vi "Boolean Update - Colors.vi"(6 "control-level":string, 10 "Bool Refnum":refnum<vi>, 11 "Material-Scheme in":refnum<class "Material-Scheme.lvclass">) -> (0 "error out":errorcluster, 1 "Array":cluster{"bg":u32, "fg":u32}[](array[cluster]), 2 "font color":u32(colorbox), 3 "Material-Scheme":refnum<class "Material-Scheme.lvclass">)   [LabVIEW 2021, in "TSC Material Theme.lvlib" / "Material-Scheme.lvclass"]
doc: "update boolean control colors\n\n<b>Code Developed By:</b>\nTechnology Service Corporation\nwww.tsc.com/atcs\n\nDeveloper:\nDaniel Coons"
uses:
  Material-Scheme.lvclass
  Material-Scheme.lvclass/Material-Scheme.ctl
panel:
  in  "error in":errorcluster
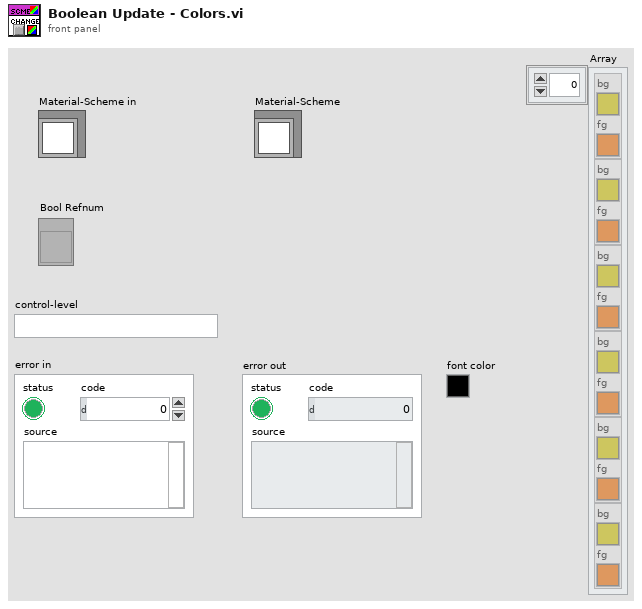
[diagram p1: front panel]
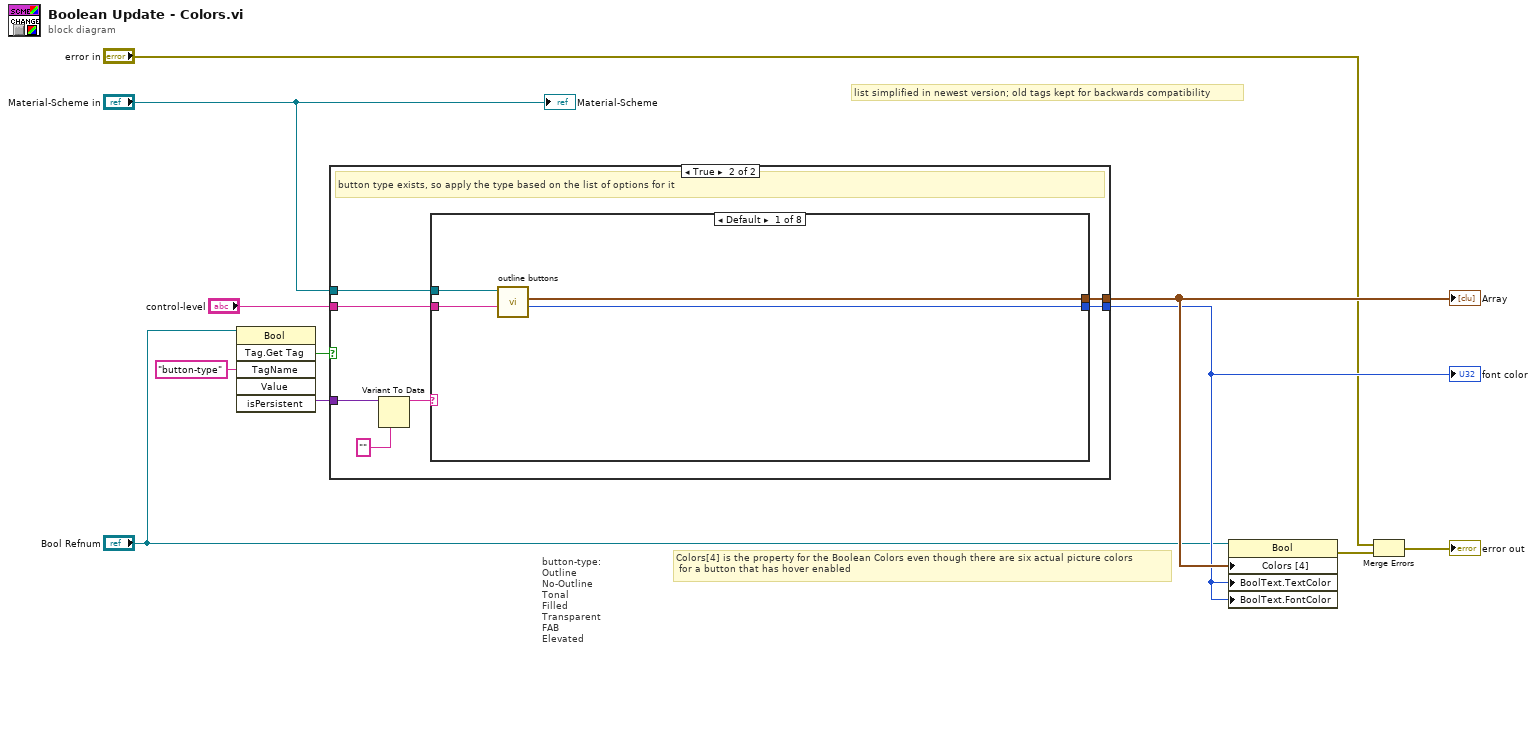
[diagram p0: block diagram]
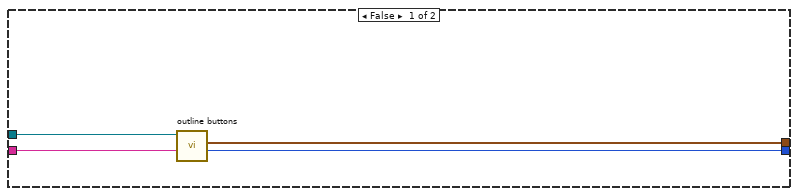
[diagram p2: hidden frame]
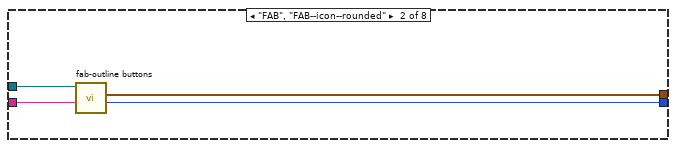
[diagram p3: hidden frame]
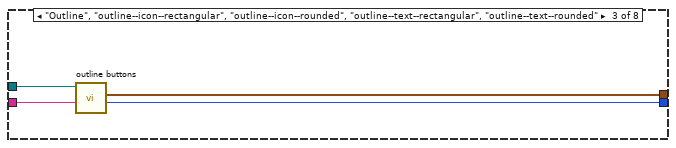
[diagram p4: hidden frame]
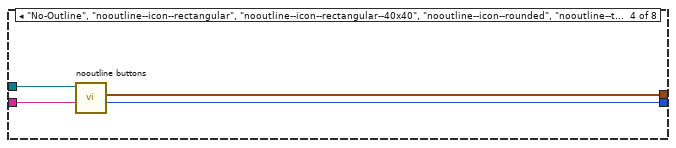
[diagram p5: hidden frame]
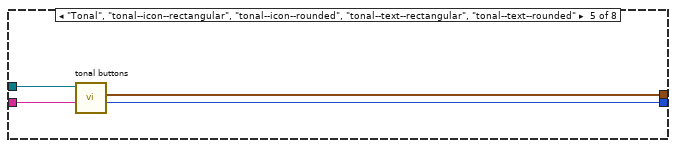
[diagram p6: hidden frame]
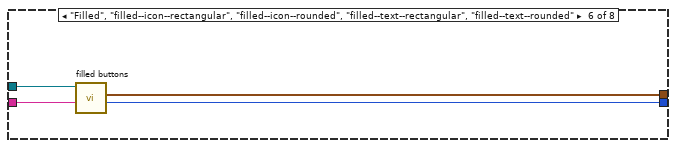
[diagram p7: hidden frame]
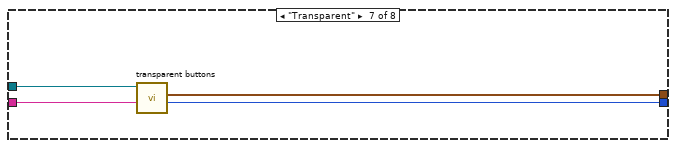
[diagram p8: hidden frame]
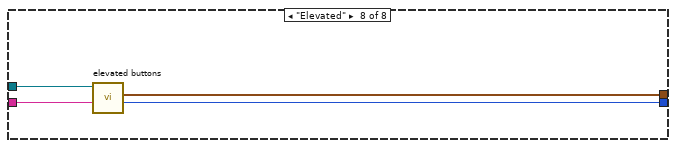
[diagram p9: hidden frame]
diagram:
  # "list simplified in newest version; old tags kept for backwards compatibility"
  # "button-type:\nOutline\nNo-Outline\nTonal\nFilled\nTransparent\nFAB\nElevated"
  # "Colors[4] is the property for the Boolean Colors even though there are six actual picture colors\n for a button that has hover enabled"
  n1 = invoke class="Bool" method="Tag.Get Tag"(reference="Bool Refnum", "TagName"="button-type" ("Tag Name")) -> ("GetTag"=w10:bool, "isPersistent"=w9:variant)  [unwired: 4 in, 4 out]
  n2 = case shown="True" w10 {
    tunnel: w9 -> [_ w22]
    tunnel: [w14 w19] -> w8
    tunnel: [w13 w18] -> w7
    tunnel: "Material-Scheme in" -> [w15 w17]
    tunnel: "control-level" -> [w12 w16]
    frame False {
      n3 = call "outline buttons.vi"("control-level"=w12, "Material-Scheme in"=w15) -> ("font color"=w13:u32, "colors array"=w14:cluster{"bg":u32, "fg":u32}[])  [unwired: 8 in]
    }
    frame True {
      # "button type exists, so apply the type based on the list of options for it"
      n4 = Variant To Data(type="", Variant=w22) -> (data=w20:string)  [unwired: 1 in, 1 out]
      n5 = case shown="Default" w20 {
        tunnel: [w26 w30 w34 w38 w42 w46 w48 w52] -> w19
        tunnel: [w25 w29 w33 w37 w41 w45 w47 w51] -> w18
        tunnel: w17 -> [w24 w28 w32 w36 w40 w44 w50 w54]
        tunnel: w16 -> [w23 w27 w31 w35 w39 w43 w49 w53]
        frame Default {
          n6 = call "outline buttons.vi"("control-level"=w23, "Material-Scheme in"=w24) -> ("font color"=w25:u32, "colors array"=w26:cluster{"bg":u32, "fg":u32}[])  [unwired: 8 in]
        }
        frame "FAB", "FAB--icon--rounded" {
          n7 = call "fab-outline buttons.vi"("control-level"=w27, "Material-Scheme in"=w28) -> ("font color"=w29:u32, "colors array"=w30:cluster{"bg":u32, "fg":u32}[])  [unwired: 8 in]
        }
        frame "Outline", "outline--icon--rectangular", "outline--icon--rounded", "outline--text--rectangular", "outline--text--rounded" {
          n8 = call "outline buttons.vi"("control-level"=w31, "Material-Scheme in"=w32) -> ("font color"=w33:u32, "colors array"=w34:cluster{"bg":u32, "fg":u32}[])  [unwired: 8 in]
        }
        frame "No-Outline", "nooutline--icon--rectangular", "nooutline--icon--rectangular--40x40", "nooutline--icon--rounded", "nooutline--text--rectangular", "nooutline--text--rounded" {
          n9 = call "nooutline buttons.vi"("control-level"=w35, "Material-Scheme in"=w36) -> ("font color"=w37:u32, "colors array"=w38:cluster{"bg":u32, "fg":u32}[])  [unwired: 8 in]
        }
        frame "Tonal", "tonal--icon--rectangular", "tonal--icon--rounded", "tonal--text--rectangular", "tonal--text--rounded" {
          n10 = call "tonal buttons.vi"("control-level"=w39, "Material-Scheme in"=w40) -> ("font color"=w41:u32, "colors array"=w42:cluster{"bg":u32, "fg":u32}[])  [unwired: 8 in]
        }
        frame "Filled", "filled--icon--rectangular", "filled--icon--rounded", "filled--text--rectangular", "filled--text--rounded" {
          n11 = call "filled buttons.vi"("control-level"=w43, "Material-Scheme in"=w44) -> ("font color"=w45:u32, "colors array"=w46:cluster{"bg":u32, "fg":u32}[])  [unwired: 8 in]
        }
        frame "Transparent" {
          n12 = call "transparent buttons.vi"("control-level"=w49, "Material-Scheme in"=w50) -> ("font color"=w47:u32, "colors array"=w48:cluster{"bg":u32, "fg":u32}[])  [unwired: 8 in]
        }
        frame "Elevated" {
          n13 = call "elevated buttons.vi"("control-level"=w53, "Material-Scheme in"=w54) -> ("font color"=w51:u32, "colors array"=w52:cluster{"bg":u32, "fg":u32}[])  [unwired: 8 in]
        }
      }
    }
  }
  "Array" <- w8
  "font color" <- w7
  n14 = property class="Bool"(reference="Bool Refnum", "Colors [4]"=w8, "BoolText.TextColor"=w7, "BoolText.FontColor"=w7) -> (error out=w3:errorcluster)  [unwired: 1 in, 1 out]
  n15 = Merge Errors("error in", w3) -> (→"error out":errorcluster)
  "Material-Scheme" <- "Material-Scheme in"
